vi "List Root Test ID.vi"(8 "error in (no error)":errorcluster, 11 "Test Executive Ref":refnum<data-value>) -> (0 "error out":errorcluster, 1 "Root IDs":string[](array[string]), 2 "Root Names":string[](array[string]), 3 "Test Executive Ref out":refnum<data-value>, 5 "Root ID":string)   [LabVIEW 2020, in "Test Executive.lvlib" / "TestExecutive Ref.lvclass"]
uses:
  <vilib>/gpm_packages/@cs/test-executive/Source/Test Executive/TestExecutive Ref/TestExecutive Ref.lvclass
  <vilib>/gpm_packages/@cs/test-executive/Source/Test Executive/ITestExecutive/ITest Executive.lvclass
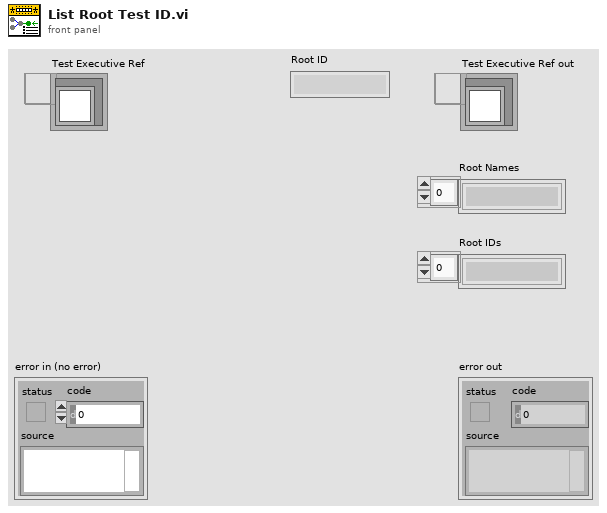
[diagram p1: front panel]
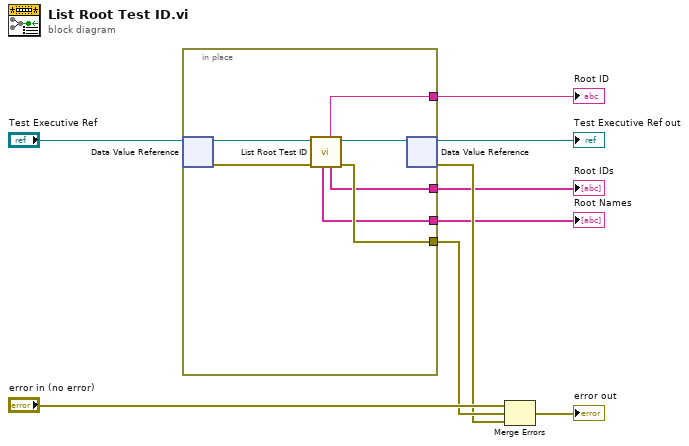
[diagram p0: block diagram]
diagram:
  n1 = in-place {
    in-place-border: [w15] -> w6
    in-place-border: [w12] -> w3
    in-place-border: [w11] -> w2
    in-place-border: [w10] -> w1
    n2 = in-place-dvr #1("Test Executive Ref") -> (w14:refnum<class "ITest Executive.lvclass">, w16:errorcluster)
    n3 = call-dynamic "List Root Test ID.vi"("error in (no error)"=w16, "ITest Executive in"=w14) -> ("error out"=w15:errorcluster, "ITest Executive out"=w13:refnum<class "ITest Executive.lvclass">, "Root IDs"=w11:string[], "Root ID"=w12:string, "Root Names"=w10:string[])  [unwired: 5 in]
    n4 = in-place-dvr #1(w13) -> (→"Test Executive Ref out":refnum<data-value>, w5:errorcluster)
  }
  "Root ID" <- w3
  "Root IDs" <- w2
  "Root Names" <- w1
  n5 = Merge Errors("error in (no error)", w6, w5) -> (→"error out":errorcluster)
